vi "LatentDirichletAllocation.vi"(8 "error in":errorcluster) -> (0 "error out":errorcluster, 3 "out":refnum<class "LatentDirichletAllocation.lvclass">)   [LabVIEW 2020]
doc: "Latent Dirichlet Allocation with online variational Bayes algorithm\n\n .. versionadded:: 0.17\n\n Read more in the :ref:`User Guide <LatentDirichletAllocation>`.\n\n Parameters\n ----------\n n_components : int, default=10\n Number of topics.\n\n .. versionchanged:: 0.19\n ``n_topics`` was renamed to ``n_components``\n\n doc_topic_prior : float, default=None\n Prior of document topic distribution `theta`. If the value is None,\n defaults to `1 / n_components`.\n In [1]_, this is called `alpha`.\n\n topic_word_prior : float, default=None\n Prior of topic word distribution `beta`. If the value is None, defaults\n to `1 / n_components`.\n In [1]_, this is called `eta`.\n\n learning_method : {'batch', 'online'}, default='batch'\n Method used to update `_component`. Only used in :meth:`fit` method.\n In general, if the data size is large, the online update will be much\n faster than the batch update.\n\n Valid options::\n\n 'batch': Batch variational Bayes method. Use all training data in\n each EM update.\n Old `components_` will be overwritten in each iteration.\n 'online': Online variational Bayes method. In each EM update, use\n mini-batch of training data to update the ``components_``\n variable incrementally. The learning rate is controlled by the\n ``learning_decay`` and the ``learning_offset`` parameters.\n\n .. versionchanged:: 0.20\n The default learning method is now ``\"batch\"``.\n\n learning_decay : float, default=0.7\n It is a parameter that control learning rate in the online learning\n method. The value should be set between (0.5, 1.0] to guarantee\n asymptotic convergence. When the value is 0.0 and batch_size is\n ``n_samples``, the update method is same as batch learning. In the\n literature, this is called kappa.\n\n learning_offset : float, default=10.\n A (positive) parameter that downweights early iterations in online\n learning. It should be greater than 1.0. In the literature, this is\n called tau_0.\n\n max_iter : int, default=10\n The maximum number of iterations.\n\n batch_size : int, default=128\n Number of documents to use in each EM iteration. Only used in online\n learning.\n\n evaluate_every : int, default=-1\n How often to evaluate perplexity. Only used in `fit` method.\n set it to 0 or negative number to not evaluate perplexity in\n training at all. Evaluating perplexity can help you check convergence\n in training process, but it will also increase total training time.\n Evaluating perplexity in every iteration might increase training time\n up to two-fold.\n\n total_samples : int, default=1e6\n Total number of documents. Only used in the :meth:`partial_fit` method.\n\n perp_tol : float, default=1e-1\n Perplexity tolerance in batch learning. Only used when\n ``evaluate_every`` is greater than 0.\n\n mean_change_tol : float, default=1e-3\n Stopping tolerance for updating document topic distribution in E-step.\n\n max_doc_update_iter : int, default=100\n Max number of iterations for updating document topic distribution in\n the E-step.\n\n n_jobs : int, default=None\n The number of jobs to use in the E-step.\n ``None`` means 1 unless in a :obj:`joblib.parallel_backend` context.\n ``-1`` means using all processors. See :term:`Glossary <n_jobs>`\n for more details.\n\n verbose : int, default=0\n Verbosity level.\n\n random_state : int, RandomState instance or None, default=None\n Pass an int for reproducible results across multiple function calls.\n See :term:`Glossary <random_state>`.\n\n Attributes\n ----------\n components_ : ndarray of shape (n_components, n_features)\n Variational parameters for topic word distribution. Since the complete\n conditional for topic word distribution is a Dirichlet,\n ``components_[i, j]`` can be viewed as pseudocount that represents the\n number of times word `j` was assigned to topic `i`.\n It can also be viewed as distribution over the words for each topic\n after normalization:\n ``model.components_ / model.components_.sum(axis=1)[:, np.newaxis]``.\n\n exp_dirichlet_component_ : ndarray of shape (n_components, n_features)\n Exponential value of expectation of log topic word distribution.\n In the literature, this is `exp(E[log(beta)])`.\n\n n_batch_iter_ : int\n Number of iterations of the EM step.\n\n n_iter_ : int\n Number of passes over the dataset.\n\n bound_ : float\n Final perplexity score on training set.\n\n doc_topic_prior_ : float\n Prior of document topic distribution `theta`. If the value is None,\n it is `1 / n_components`.\n\n random_state_ : RandomState instance\n RandomState instance that is generated either from a seed, the random\n number generator or by `np.random`.\n\n topic_word_prior_ : float\n Prior of topic word distribution `beta`. If the value is None, it is\n `1 / n_components`.\n\n \nAvailable methods:\nFit\nFit Transform\nTransform\nGet Attributes\nGet Params\nSet Params"
uses:
  LatentDirichletAllocation.lvclass
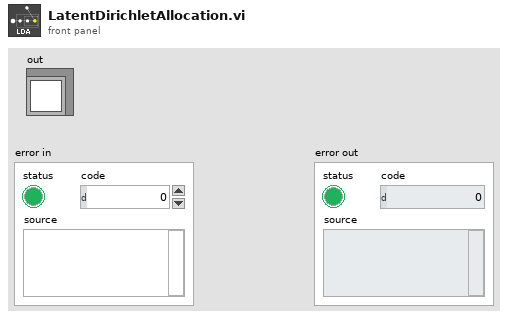
[diagram p1: front panel]
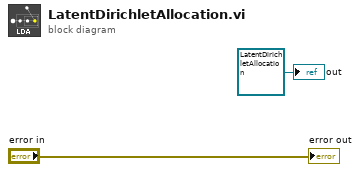
[diagram p0: block diagram]
diagram:
  "out" <- refnum<class "LatentDirichletAllocation.lvclass"> refnum ("model")
  "error out" <- "error in"
